vi "Configure Questionable Ntransition Value.vi"(8 "error in (no error)":errorcluster, 10 "Value(0)":u32 step=1, 11 "VISA resource name":refnum<visa-resource-name>) -> (0 "error out":errorcluster, 3 "VISA resource name out":refnum<visa-resource-name>)   [LabVIEW 2015, in "IT6000C.lvlib"]
doc: "Sets the value of the NTR (negative transition) register.These registers act as polar filters between the problem condition and the problem event registers.When the bit in the NTR register is set to 1, the 1-0 conversion of the corresponding bit in the problem condition register causes that bit to be set in the problem event register.STATus: can be set to PRESet PTR all a bit in a register, and remove NTR all the bits in the register.\n1: if the same bit in the NTR and PTR registers is set to 1, any conversion of that bit in the problem condition register sets the corresponding bit in the problem event register.\n2: if the same bit in the NTR and PTR registers is set to 0, any conversion of that bit in the problem condition register will not set the corresponding bit in the problem event register.\n3: the return value is the sum of all binary weighted bits enabled in the register.\n\n<b>Value</b>\nRange:0-0x7fffffff"
uses:
  <instrlib>/IT6000C/IT6000C.lvlib
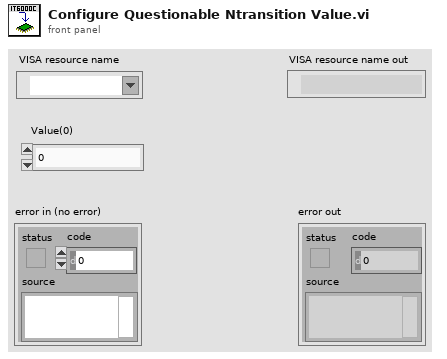
[diagram p1: front panel]
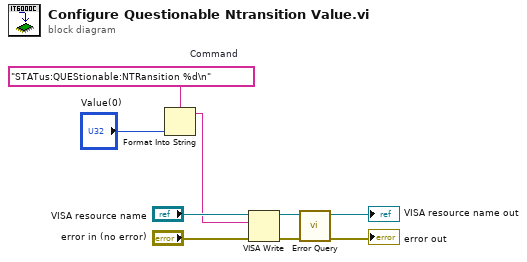
[diagram p0: block diagram]
diagram:
  w3 = "STATus:QUEStionable:NTRansition %d\n"  # Command
  n1 = Format Into String(format string=w3, "Value(0)") -> (resulting string=w1:string)  [unwired: 2 in, 1 out]
  n2 = VISA Write(VISA resource name="VISA resource name", write buffer=w1, error in (no error)="error in (no error)") -> (VISA resource name out=w6:refnum<visa-resource-name>, error out=w7:errorcluster)  [unwired: 1 out]
  n3 = call <instrlib>:"Error Query.vi"("error in (no error)"=w7, "VISA resource name"=w6) -> ("error out"=→"error out":errorcluster, "VISA resource name out"=→"VISA resource name out":refnum<visa-resource-name>)  [unwired: 6 in, 2 out]
